vi "Toolbar Faacade.vi"(0 "Data In":T5, 2 "Display State In":T2={"Buttons Displayed"=0, "Button States"=[], "Button Size"=0, "Button Style"=enum."Classic", "Active Button"=0, "Force Regen?"=FALSE, "Tip String Ref"=refnum}, 3 "Container State":T4) -> (6 "Data Out":T5, 7 "Display State Out":T2={"Buttons Displayed"=0, "Button States"=[], "Button Size"=0, "Button Style"=enum."Classic", "Active Button"=0, "Force Regen?"=FALSE, "Tip String Ref"=refnum}, 8 "Action":T1)   [LabVIEW 2012, in "Toolbar.xctl"]
doc: "The business end of the XControl..."
uses:
  Toolbar.xctl
  Toolbar Data.ctl
  Button_Class/Type Defs/Button Events.ctl
  <vilib>/_xctls/Container State.ctl
  Toolbar State.ctl
  Button_Class/Button.lvclass
  Button_Class/Type Defs/Button Style.ctl
  <vilib>/_xctls/Action.ctl
  Button_Class/Type Defs/Button Status.ctl
  <vilib>/_xctls/XControlSupport.lvlib
panel:
  out "Display":picture[](array[picture])
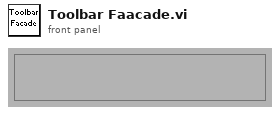
[diagram p1: front panel]
types:
  T1 = typedef "XControlSupport.lvlib/Action.ctl" = cluster{"Data Changed?":bool, "State Changed?":bool, "Action Name":string}
  T2 = typedef "Toolbar.xctl/Toolbar State.ctl" = cluster{"Buttons Displayed":i32, "Button States":refnum<class "Button.lvclass">[], "Button Size":i32, "Button Style":T3, "Active Button":i32, "Force Regen?":bool, "Tip String Ref":refnum<vi>}
  T3 = typedef "Button.lvclass/Button Style.ctl" = enum16{"System", "Modern", "Classic", "Rounded", "Silver", "Ni Theme", "Metallic"}
  T4 = typedef "XControlSupport.lvlib/Container State.ctl" = cluster{"Indicator?":bool, "Run Mode?":bool, " Refnum":refnum<vi>}
  T5 = typedef "Toolbar.xctl/Toolbar Data.ctl" = cluster{"Index":i32, "Type":T6}
  T6 = typedef "Button.lvclass/Button Events.ctl" = enum16{"Click", "Latch", "Unlatch"}
  T7 = typedef "Button.lvclass/Button Status.ctl" = enum16{"Off", "Hover", "On", "Disabled"}
  T8 = enum16{"NoButton", "Left Button", "Right Button", "Middle Button"}
  T9 = typedef "LVPoint32TypeDef.ctl" = cluster{"Horizontal":i32, "Vertical":i32}
  T10 = typedef "LVRectTypeDef.ctl" = cluster{"Left":i16, "Top":i16, "Right":i16, "Bottom":i16}
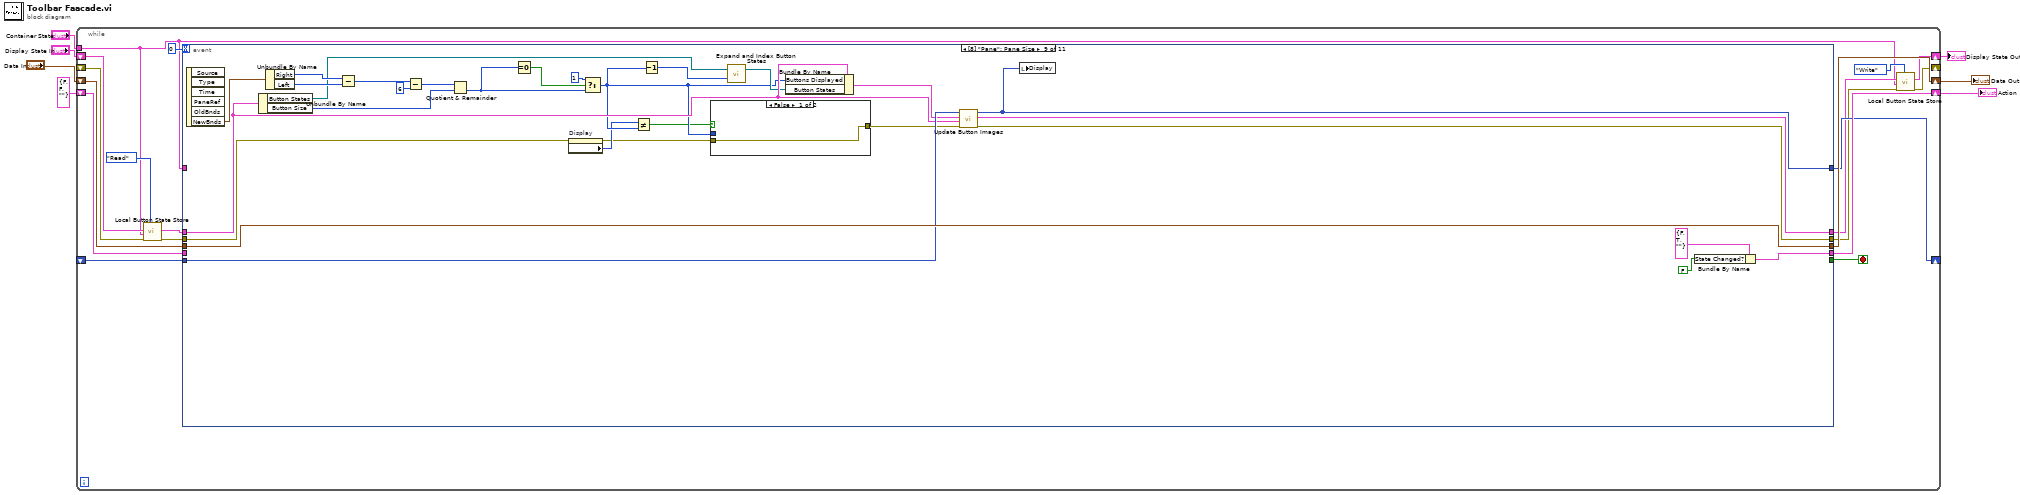
[diagram p0: block diagram]
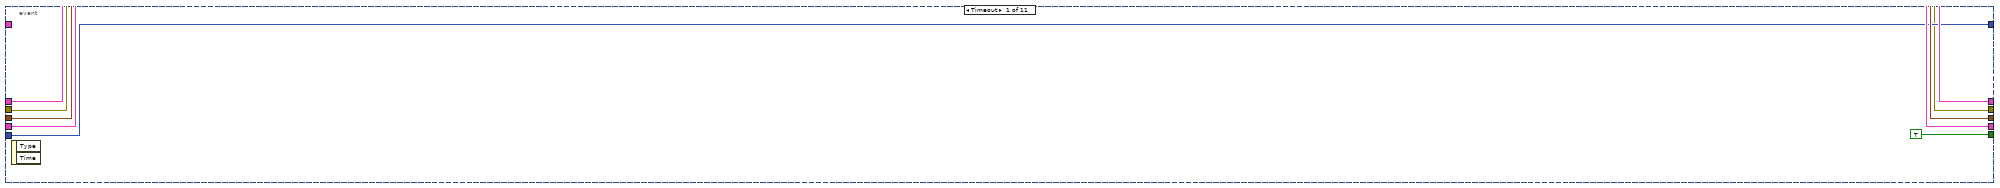
[diagram p2: hidden frame]
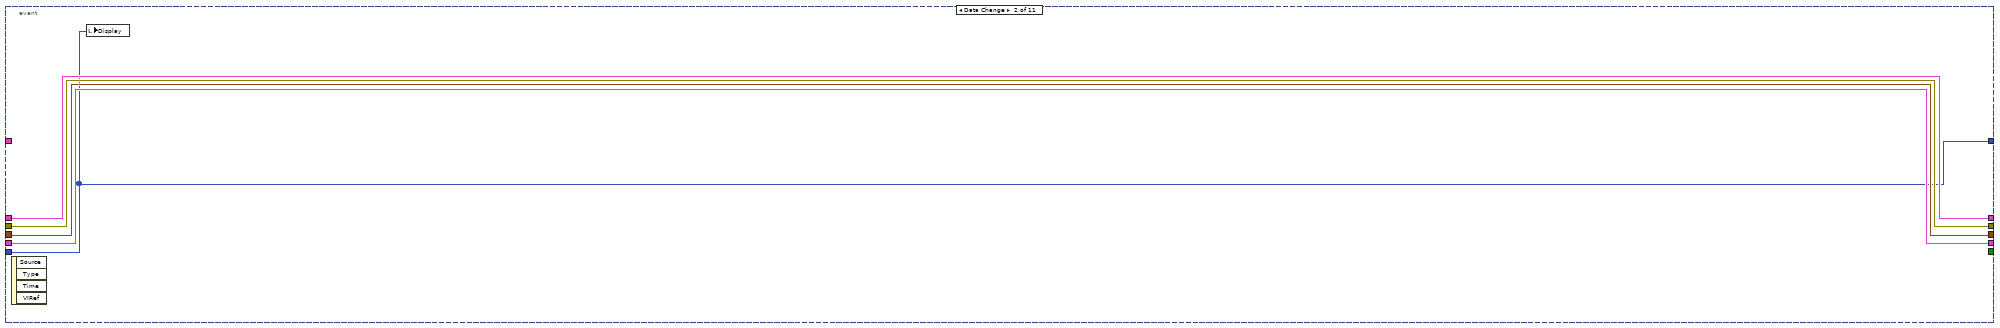
[diagram p3: hidden frame]
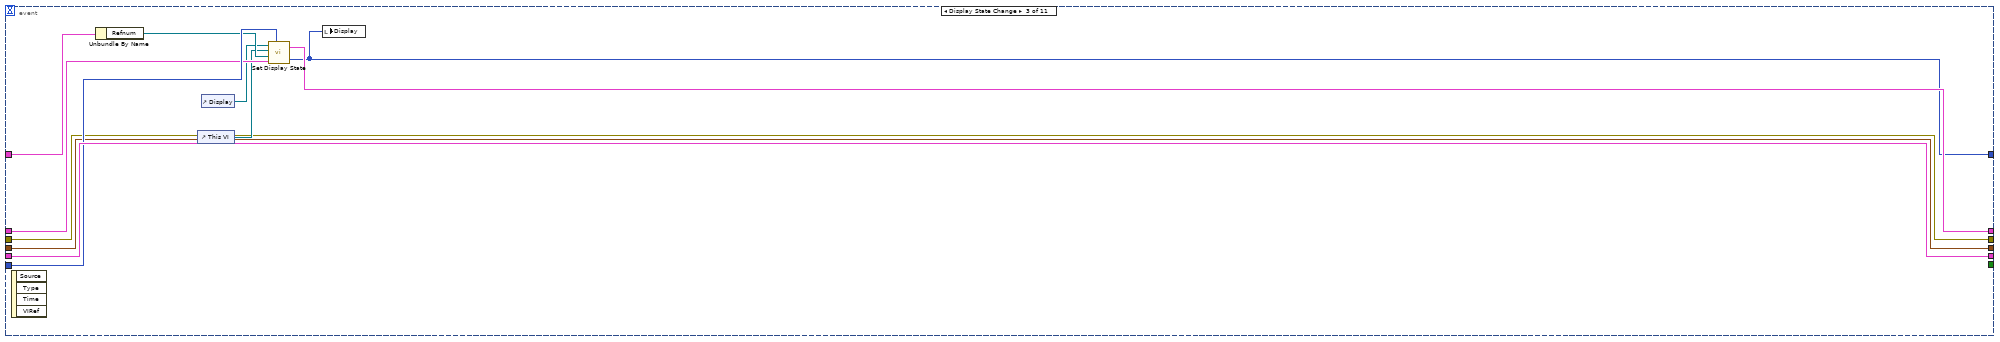
[diagram p4: hidden frame]
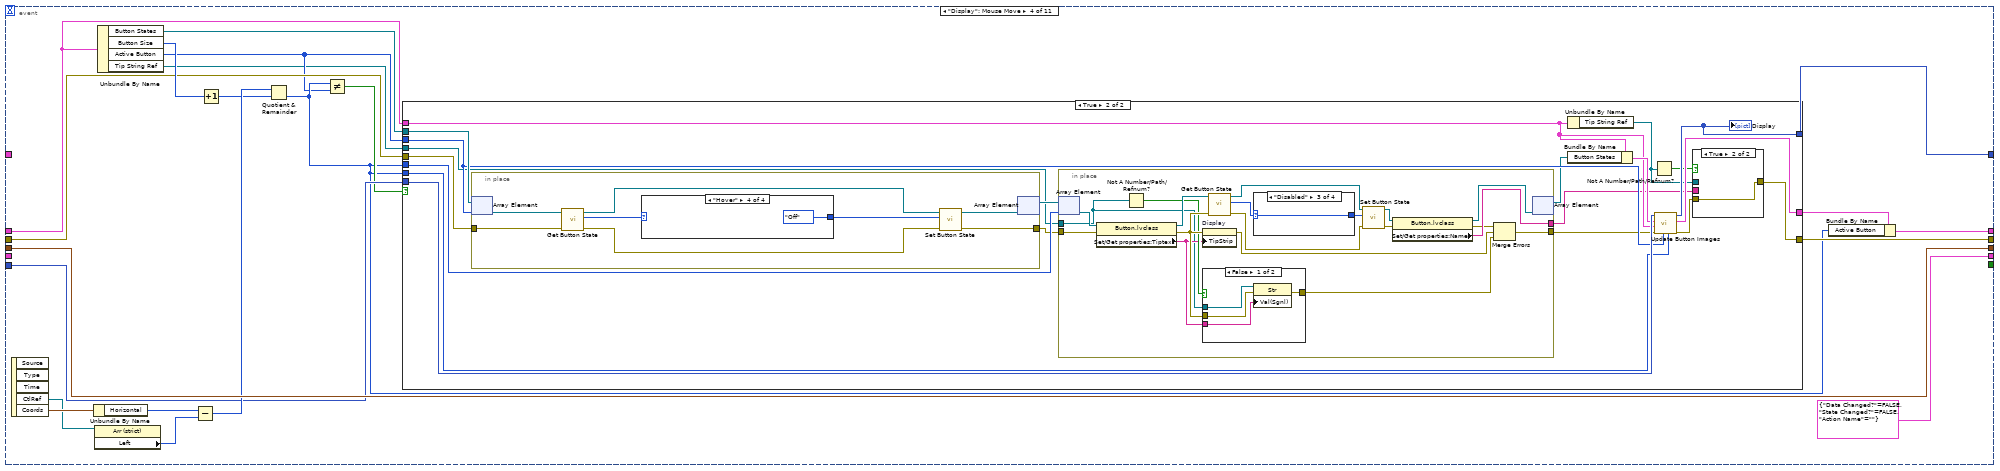
[diagram p5: hidden frame]
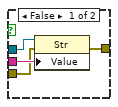
[diagram p7: hidden frame]
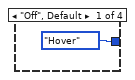
[diagram p9: hidden frame]
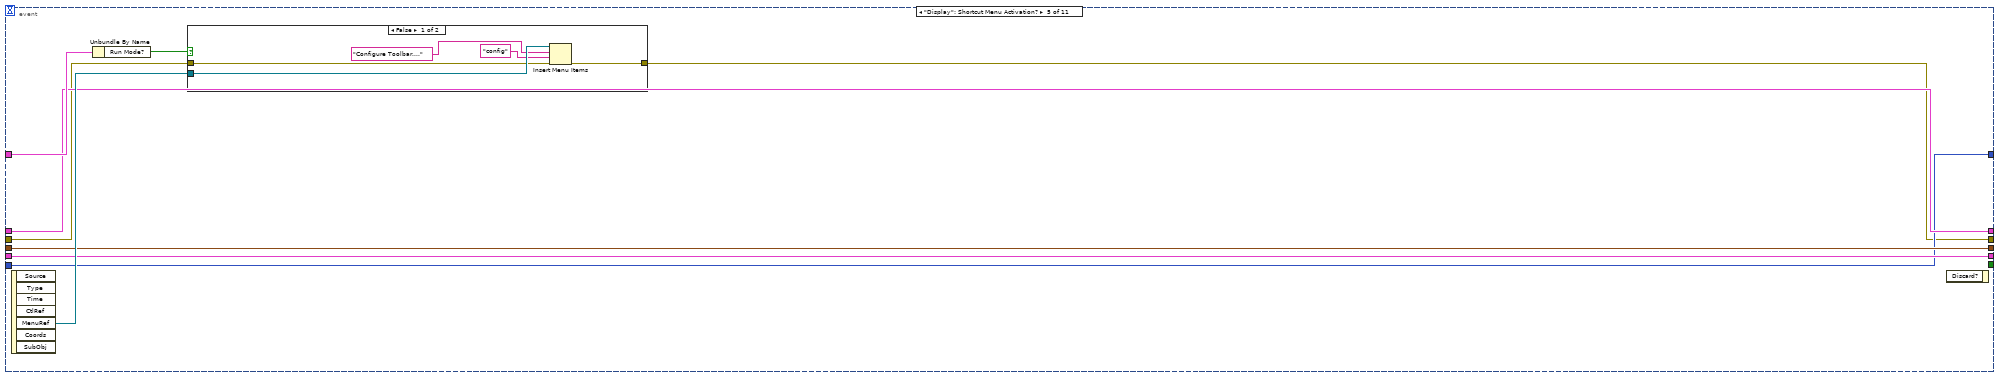
[diagram p15: hidden frame]
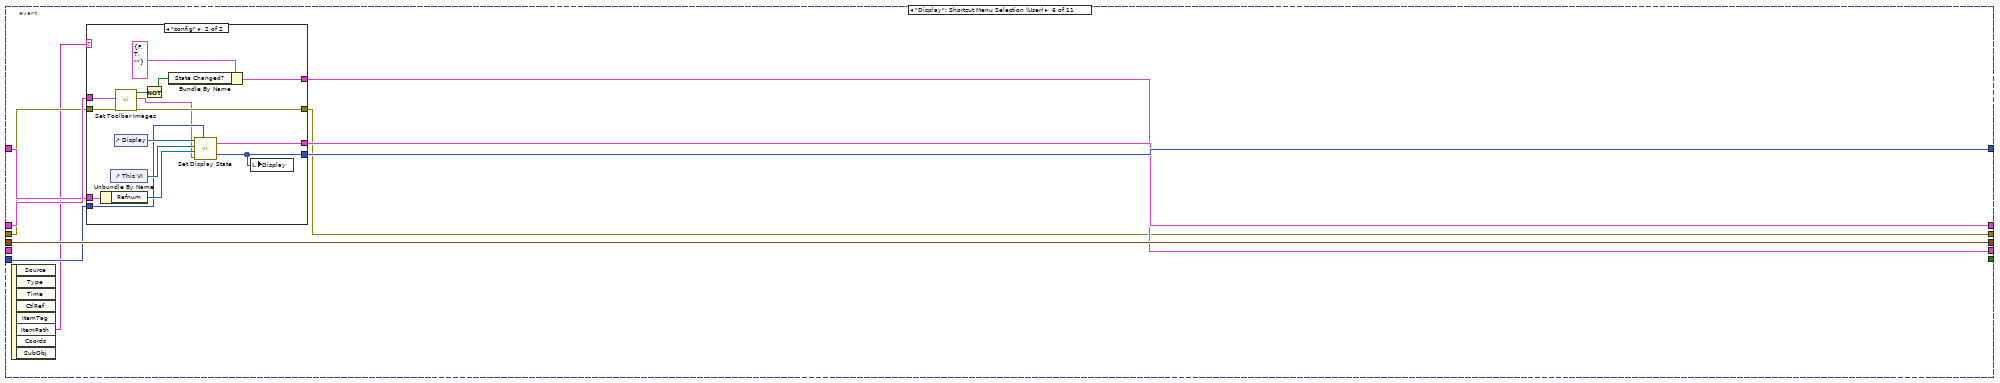
[diagram p17: hidden frame]
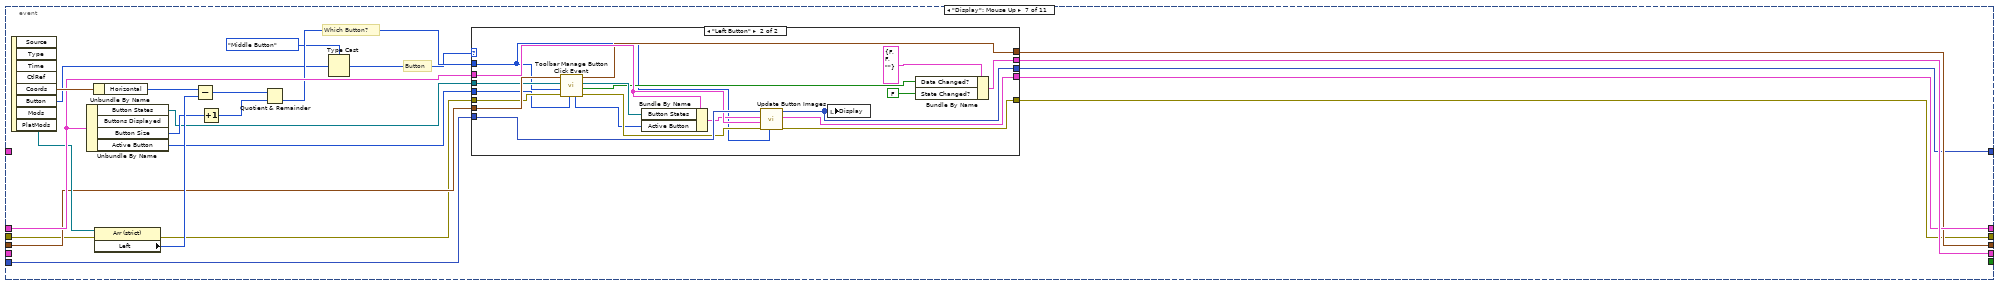
[diagram p19: hidden frame]
diagram:
  n1 = while {
    shift-right: [w8] -> w4
    shift-left: "Display State In" -> [w12]
    tunnel: "Container State" -> [w10]
    shift-right: [w23] -> w7
    shift-left: "Data In" -> [w24]
    shift-right: [w21] -> w2
    shift-left: T1 {"Data Changed?"=FALSE, "State Changed?"=FALSE, "Action Name"=""} ("Action") -> [w22]
    shift-right: [w20] -> _
    shift-left: _ -> [w19]
    shift-right: [w15] -> _
    shift-left: _ -> [w14]
    stop <- w26 stop-if-true
    n2 = call "Local Button State Store.vi"("Operation"=enum16{"Read", "Write"}."Read", "error in (no error)"=w14, "Container State"=w10, "Display State In"=w12) -> ("error out"=w13:errorcluster, "Display State Out"=w9:T2)  [unwired: 6 out]
    n3 = event shown="[8] \"Pane\": Pane Size" {
      selector: _ -> [_ _ _ _ _ _ _ _ _ _ _]
      dyn-events: _ -> [_ _ _ _ _ _ _ _ _ _ _]
      timeout: 0 -> [_ _ _ _ _ _ _ _ _ _ _]
      tunnel: w9 -> [w30 w36 w44 w53 w142 w161 w200 w230 w272 w295 w305]
      tunnel: [w30 w36 w41 w52 w142 w158 w195 w235 w270 w295 w304] -> w11
      tunnel: [TRUE _ _ _ _ _ _ _ _ _ _] -> w26
      tunnel: w10 -> [_ _ w46 _ w145 w157 _ _ _ w296 w311]
      tunnel: w24 -> [w29 w37 w39 w66 w143 w162 w193 w237 w278 w294 w310]
      tunnel: [w29 w37 w39 w66 w143 w162 w192 w237 w278 w294 w310] -> w23
      tunnel: [w31 w35 w48 T1 {"Data Changed?"=FALSE, "State Changed?"=FALSE, "Action Name"=""} ("Action") w141 w156 w203 T1 {"Data Changed?"=FALSE, "State Changed?"=FALSE, "Action Name"=""} ("Action") w263 w293 w309] -> w21
      tunnel: w22 -> [w31 w35 w48 _ w141 _ _ _ _ w293 w309]
      tunnel: [w28 w33 w38 w62 w140 w159 w191 w227 w256 w292 w307] -> w20
      tunnel: w19 -> [w28 w33 w47 w61 w140 w160 w190 w236 w276 w292 w308]
      tunnel: [w27 w34 w40 w57 w139 w154 w185 w232 w260 w288 w302] -> w16
      tunnel: w13 -> [w27 w34 w40 w56 w138 w155 w184 w234 w257 w289 w303]
      event Timeout {
        n4 = event-data() -> ()  [unwired: 3 out]
      }
      event Data Change {
        n5 = event-data() -> ()  [unwired: 5 out]
        n6 = local write "Display"(w33) -> ()
      }
      event Display State Change {
        n7 = event-data() -> ()  [unwired: 5 out]
        n8 = Unbundle By Name(w46) -> ("Refnum"=w45:refnum<vi>)
        n9 = control-ref of="This VI"() -> (w43:refnum<vi>)
        n10 = control-ref of="Display"() -> (w42:refnum<vi>)
        n11 = call "Set Display State.vi"("Picture Array Refnum"=w42, "Facade Vi Refnum"=w43, "Container Refnum"=w45, "Display State In"=w44, "Display"=w47) -> ("State Out"=w41:T2, "Images Out"=w38:picture[])
        n12 = local write "Display"(w38) -> ()
      }
      event "Display": Mouse Move {
        n13 = event-data() -> ("CtlRef"=w65:refnum<vi>, "Coords"=w68:T9)  [unwired: 4 out]
        n14 = Unbundle By Name(w68) -> ("Horizontal"=w67:i32)
        n15 = property class="Arr (strict)"(reference=w65) -> ("Left"=w63:i32)  [unwired: 1 in, 2 out]
        n16 = Unbundle By Name(w53) -> ("Button States"=w55:refnum<class "Button.lvclass">[], "Button Size"=w59:i32, "Active Button"=w50:i32, "Tip String Ref"=w49:refnum<vi>)
        n17 = Subtract(x=w67, y=w63) -> (x-y=w64:i32)
        n18 = Increment(x=w59) -> (x+1=w58:i32)
        n19 = Quotient & Remainder(x=w64, y=w58) -> (floor(x/y)=w51:i32)  [unwired: 1 out]
        n20 = Not Equal?(x=w51, y=w50) -> (x != y?=w54:bool)
        n21 = case shown="True" w54 {
          tunnel: [w72 w80] -> w62
          tunnel: w61 -> [w72 w92]
          tunnel: w53 -> [w71 w79]
          tunnel: [w71 w90] -> w60
          tunnel: [w70 w74] -> w57
          tunnel: w56 -> [w70 w86]
          tunnel: w55 -> [_ w88]
          tunnel: w51 -> [_ w84]
          tunnel: w50 -> [_ w87]
          tunnel: w51 -> [_ w89]
          tunnel: w49 -> [_ w73]
          frame False {
          }
          frame True {
            n22 = in-place {
              in-place-border: w86 -> [w129]
              in-place-border: [w126] -> w83
              n23 = in-place-array #1(w88, w87) -> (w133:refnum<class "Button.lvclass">)
              n24 = call-dynamic "Get Button State.vi"("error in (no error)"=w129, "Button in"=w133) -> ("error out"=w128:errorcluster, "State"=w131:T7, "Button out"=w132:refnum<class "Button.lvclass">)  [unwired: 1 in, 6 out]
              n25 = case shown="\"Hover\"" w131 {
                selector: w131 -> [w134 w135 w136 _]
                tunnel: [w134 w135 w136 Button_Status."Off" ("State")] -> w130
                frame "Off", Default {
                }
                frame "On" {
                }
                frame "Disabled" {
                }
                frame "Hover" {
                }
              }
              n26 = call-dynamic "Set Button State.vi"("error in (no error)"=w128, "State"=w130, "Button in"=w132) -> ("error out"=w126:errorcluster, "Button out"=w127:refnum<class "Button.lvclass">)  [unwired: 7 out]
              n27 = in-place-array #1(w127) -> (w85:refnum<class "Button.lvclass">[])  [unwired: 1 out]
            }
            n28 = in-place {
              in-place-border: w83 -> [w107]
              in-place-border: [w99] -> w81
              in-place-border: [w109] -> w76
              in-place-border: w73 -> [w98]
              n29 = in-place-array #2(w85, w84) -> (w116:refnum<class "Button.lvclass">)
              n30 = property class="Button.lvclass"(reference=w116, error in=w107) -> (reference out=w108:refnum<class "Button.lvclass">, error out=w106:errorcluster, "Set/Get properties:Tiptext"=w104:string)
              n31 = Not A Number/Path/Refnum?(number/path/refnum=w98) -> (NaN/Path/Refnum?=w105:bool)
              n32 = property on="Display" class="Arr (strict)"(error in=w106, "TipStrip"=w104) -> (error out=w101:errorcluster)  [unwired: 1 in, 1 out]
              n33 = case shown="False" w105 {
                tunnel: w106 -> [w120 w121]
                tunnel: w104 -> [w119 _]
                tunnel: [w118 w121] -> w100
                tunnel: w98 -> [w117 _]
                frame False {
                  n34 = property class="Str"(reference=w117, error in=w120, "Val(Sgnl)"=w119) -> (error out=w118:errorcluster)  [unwired: 1 out]
                }
                frame True {
                }
              }
              n35 = call-dynamic "Get Button State.vi"("error in (no error)"=w106, "Button in"=w108) -> ("error out"=w112:errorcluster, "State"=w114:T7, "Button out"=w115:refnum<class "Button.lvclass">)  [unwired: 1 in, 6 out]
              n36 = case shown="\"Disabled\"" w114 {
                selector: w114 -> [_ w123 w124 w125]
                tunnel: [Button_Status."Hover" ("State") w123 w124 w125] -> w113
                frame "Off", Default {
                }
                frame "On" {
                }
                frame "Disabled" {
                }
                frame "Hover" {
                }
              }
              n37 = call-dynamic "Set Button State.vi"("error in (no error)"=w112, "State"=w113, "Button in"=w115) -> ("error out"=w103:errorcluster, "Button out"=w111:refnum<class "Button.lvclass">)  [unwired: 7 out]
              n38 = property class="Button.lvclass"(reference=w111, error in=w103) -> (reference out=w110:refnum<class "Button.lvclass">, error out=w102:errorcluster, "Set/Get properties:Name"=w109:string)
              n39 = Merge Errors(w102, w101, w100) -> (w99:errorcluster)
              n40 = in-place-array #2(w110) -> (w82:refnum<class "Button.lvclass">[])  [unwired: 1 out]
            }
            n41 = Unbundle By Name(w79) -> ("Tip String Ref"=w77:refnum<vi>)
            n42 = Bundle By Name(cluster=w79, "Button States"=w82) -> (w91:T2)
            n43 = Not A Number/Path/Refnum?(number/path/refnum=w77) -> (NaN/Path/Refnum?=w78:bool)
            n44 = call "Update Button Images.vi"("New Index"=w89, "Old Index"=w87, "error in (no error)"=w81, "Old State"=w79, "New State"=w91, "Images In"=w92) -> ("error out"=w75:errorcluster, "State Out"=w90:T2, "Images Out"=w80:picture[])  [unwired: 1 in, 2 out]
            "Display" <- w80
            n45 = case shown="True" w78 {
              tunnel: w77 -> [w96 _]
              tunnel: w76 -> [w95 _]
              tunnel: w75 -> [w94 w97]
              tunnel: [w93 w97] -> w74
              frame False {
                n46 = property class="Str"(reference=w96, error in=w94, "Value"=w95) -> (error out=w93:errorcluster)  [unwired: 1 out]
              }
              frame True {
              }
            }
          }
        }
        n47 = Bundle By Name(cluster=w60, "Active Button"=w51) -> (w52:T2)
      }
      event "Display": Shortcut Menu Activation? {
        n48 = event-data() -> ("MenuRef"=w146:refnum<k9>)  [unwired: 7 out]
        n49 = Unbundle By Name(w145) -> ("Run Mode?"=w144:bool)
        n50 = case shown="False" w144 {
          tunnel: w146 -> [w151 _]
          tunnel: [w148 w152] -> w139
          tunnel: w138 -> [w147 w152]
          frame False {
            n51 = Insert Menu Items(6:w147, 7:"config" ("item tags"), 8:"Configure Toolbar....", 9:w151) -> (0:w148:errorcluster)  [unwired: 4 out]
          }
          frame True {
          }
        }
        n52 = event-data() -> ()  [unwired: 1 in, 2 out]
      }
      event "Display": Shortcut Menu Selection (User) {
        n53 = event-data() -> ("ItemPath"=w153:string)  [unwired: 8 out]
        n54 = case shown="\"config\"" w153 {
          tunnel: w161 -> [w165 w179]
          tunnel: w160 -> [w163 w171]
          tunnel: [w163 w172] -> w159
          tunnel: [w165 w176] -> w158
          tunnel: w157 -> [_ w175]
          tunnel: [_ w173] -> w156
          tunnel: w155 -> [w164 w170]
          tunnel: [w164 w169] -> w154
          frame "False", Default {
          }
          frame "config" {
            n55 = Unbundle By Name(w175) -> ("Refnum"=w174:refnum<vi>)
            n56 = control-ref of="This VI"() -> (w178:refnum<vi>)
            n57 = control-ref of="Display"() -> (w177:refnum<vi>)
            n58 = call "Set Toolbar Images.vi"("error in (no error)"=w170, "State"=w179) -> ("error out"=w169:errorcluster, "State Out"=w166:T2, "Cancelled?"=w168:bool)  [unwired: 7 out]
            n59 = Not(x=w168) -> (.not. x?=w167:bool)
            n60 = Bundle By Name(cluster=T1 {"Data Changed?"=FALSE, "State Changed?"=TRUE, "Action Name"=""} ("Action"), "State Changed?"=w167) -> (w173:T1)
            n61 = call "Set Display State.vi"("Picture Array Refnum"=w177, "Facade Vi Refnum"=w178, "Container Refnum"=w174, "Display State In"=w166, "Display"=w171) -> ("State Out"=w176:T2, "Images Out"=w172:picture[])
            n62 = local write "Display"(w172) -> ()
          }
        }
      }
      event "Display": Mouse Up {
        # "Which Button?"
        # "Button"
        n63 = event-data() -> ("CtlRef"=w198:refnum<vi>, "Coords"=w202:T9, "Button"=w194:u16)  [unwired: 6 out]
        n64 = Unbundle By Name(w200) -> ("Button States"=w181:refnum<class "Button.lvclass">[], "Button Size"=w189:i32, "Active Button"=w182:i32)  [unwired: 1 out]
        n65 = Unbundle By Name(w202) -> ("Horizontal"=w201:i32)
        n66 = property class="Arr (strict)"(reference=w198, error in=w184) -> (error out=w183:errorcluster, "Left"=w196:i32)  [unwired: 1 out]
        n67 = Subtract(x=w201, y=w196) -> (x-y=w197:i32)
        n68 = Increment(x=w189) -> (x+1=w188:i32)
        n69 = Quotient & Remainder(x=w197, y=w188) -> (floor(x/y)=w199:i32)  [unwired: 1 out]
        n70 = Type Cast(type=T8."Middle Button", x=w194) -> (*(type *) &x=w187:T8)
        n71 = case shown="\"Left Button\"" w187 {
          tunnel: [_ w224] -> w203
          tunnel: w181 -> [_ w214]
          tunnel: w200 -> [w207 w221]
          tunnel: w199 -> [_ w211]
          tunnel: [w207 w219] -> w195
          tunnel: w193 -> [w206 w226]
          tunnel: [w206 w215] -> w192
          tunnel: [w205 w208] -> w191
          tunnel: w190 -> [w205 w222]
          tunnel: [w204 w217] -> w185
          tunnel: w183 -> [w204 w216]
          tunnel: w182 -> [_ w210]
          frame "NoButton", Default {
          }
          frame "Left Button" {
            n72 = call "Toolbar Manage Button Click Event.vi"("Index In"=w210, "error in (no Error)"=w216, "Button Index"=w211, "Button States In"=w214, "Data In"=w226) -> ("error out"=w218:errorcluster, "Data Changed ?"=w212:bool, "Button States Out"=w213:refnum<class "Button.lvclass">[], "Data Out"=w215:T5, "Index Out"=w209:i32)  [unwired: 2 out]
            n73 = Bundle By Name(cluster=w221, "Button States"=w213, "Active Button"=w209) -> (w220:T2)
            n74 = call "Update Button Images.vi"("Old Index"=w211, "error in (no error)"=w218, "Old State"=w221, "New State"=w220, "Images In"=w222) -> ("error out"=w217:errorcluster, "State Out"=w219:T2, "Images Out"=w208:picture[])  [unwired: 2 in, 2 out]
            n75 = local write "Display"(w208) -> ()
            n76 = Bundle By Name(cluster=T1 {"Data Changed?"=FALSE, "State Changed?"=FALSE, "Action Name"=""} ("Action"), "Data Changed?"=w212, "State Changed?"=FALSE) -> (w224:T1)
          }
        }
      }
      event "Display": Mouse Leave {
        n77 = event-data() -> ()  [unwired: 5 out]
        n78 = in-place {
          in-place-border: w230 -> [_]
          in-place-border: w234 -> [w244]
          in-place-border: [w243] -> w233
          in-place-border: [w239] -> w231
          w239 = -1
          n79 = in-place-cluster #3(w230) -> ("Button States"=w242:refnum<class "Button.lvclass">[], "Active Button"=w241:i32)
          n80 = in-place {
            in-place-border: w244 -> [w252]
            in-place-border: [w251] -> w243
            n81 = in-place-array #4(w242, w241) -> (w246:refnum<class "Button.lvclass">)
            n82 = call-dynamic "Get Button State.vi"("error in (no error)"=w252, "Button in"=w246) -> ("error out"=w247:errorcluster, "State"=w248:T7, "Button out"=w249:refnum<class "Button.lvclass">)  [unwired: 7 out]
            n83 = case shown="\"Hover\"" w248 {
              selector: w248 -> [w253 _]
              tunnel: [w253 Button_Status."Off" ("State")] -> w250
              frame "Off", Default {
              }
              frame "Hover" {
              }
            }
            n84 = call-dynamic "Set Button State.vi"("error in (no error)"=w247, "State"=w250, "Button in"=w249) -> ("error out"=w251:errorcluster, "Button out"=w245:refnum<class "Button.lvclass">)  [unwired: 7 out]
            n85 = in-place-array #4(w245) -> (w240:refnum<class "Button.lvclass">[])  [unwired: 1 out]
          }
          n86 = in-place-cluster #3("Button States"=w240, "Active Button"=w239) -> (w229:T2)
        }
        n87 = call "Update Button Images.vi"("New Index"=w231, "Force Regen"=FALSE, "error in (no error)"=w233, "Old State"=w230, "New State"=w229, "Images In"=w236) -> ("error out"=w232:errorcluster, "State Out"=w235:T2, "Images Out"=w227:picture[])  [unwired: 1 in, 2 out]
        n88 = local write "Display"(w227) -> ()
      }
      event Pane Size {
        n89 = event-data() -> ("NewBnds"=w264:T10)  [unwired: 6 out]
        n90 = Unbundle By Name(w272) -> ("Button States"=w255:refnum<class "Button.lvclass">[], "Button Size"=w269:i32)
        n91 = Unbundle By Name(w264) -> ("Right"=w283:i16, "Left"=w282:i16)
        n92 = Subtract(x=w283, y=w282) -> (x-y=w274:i16)
        n93 = Subtract(x=w274, y=i16 6) -> (x-y=w275:i16)
        n94 = Quotient & Remainder(x=w275, y=w269) -> (floor(x/y)=w281:i32)  [unwired: 1 out]
        n95 = Equal To 0?(x=w281) -> (x = 0?=w277:bool)
        n96 = property on="Display" class="Arr (strict)"(error in=w257) -> (error out=w258:errorcluster, "Number of Columns"=w265:u32)  [unwired: 1 in, 1 out]
        n97 = Select(t=i16 1, s=w277, f=w281) -> (s? t:f=w266:i32)
        n98 = Not Equal?(x=w265, y=w266) -> (x != y?=w262:bool)
        n99 = Decrement(x=w266) -> (x-1=w267:i32)
        n100 = case shown="False" w262 {
          tunnel: w266 -> [_ w287]
          tunnel: [w284 w286] -> w259
          tunnel: w258 -> [w284 w285]
          frame False {
          }
          frame True {
            n101 = property on="Display" class="Arr (strict)"(error in=w285, "Number of Columns"=w287) -> (error out=w286:errorcluster)  [unwired: 1 in, 1 out]
          }
        }
        n102 = call "Expand and Index Button States.vi"("Button Index"=w267, "Button States"=w255) -> ("Button States Out"=w268:refnum<class "Button.lvclass">[])  [unwired: 1 out]
        n103 = Bundle By Name(cluster=w272, "Buttons Displayed"=w266, "Button States"=w268) -> (w271:T2)
        n104 = call "Update Button Images.vi"("error in (no error)"=w259, "Old State"=w272, "New State"=w271, "Images In"=w276) -> ("error out"=w260:errorcluster, "State Out"=w270:T2, "Images Out"=w256:picture[])  [unwired: 3 in, 2 out]
        n105 = local write "Display"(w256) -> ()
        n106 = Bundle By Name(cluster=T1 {"Data Changed?"=FALSE, "State Changed?"=TRUE, "Action Name"=""} ("Action"), "State Changed?"=FALSE) -> (w263:T1)
      }
      event Direction Change {
        n107 = event-data() -> ()  [unwired: 5 out]
        n108 = Unbundle By Name(w296) -> ("Indicator?"=w290:bool, "Refnum"=w291:refnum<vi>)
        n109 = case shown="True" w290 {
          tunnel: w291 -> [_ w301]
          tunnel: w289 -> [w297 w299]
          tunnel: [w297 w298] -> w288
          frame False {
          }
          frame True {
            # "The direction of the XControl changed from a control to an indicator or vice versa. Update the appearance accordingly."
            n110 = property class="Ctl"(reference=w301, error in=w299, "Indicator"=FALSE) -> (error out=w298:errorcluster)  [unwired: 1 out]
          }
        }
      }
      event Exec State Change {
        n111 = event-data() -> ()  [unwired: 5 out]
        n112 = Unbundle By Name(w311) -> ("Run Mode?"=w306:bool)
        n113 = call "Update Button Images.vi"("Force Regen"=w306, "error in (no error)"=w303, "Old State"=w305, "New State"=w305, "Images In"=w308) -> ("error out"=w302:errorcluster, "State Out"=w304:T2, "Images Out"=w307:picture[])  [unwired: 2 in, 2 out]
        n114 = local write "Display"(w307) -> ()
      }
    }
    n115 = call "Local Button State Store.vi"("Operation"=enum16{"Read", "Write"}."Write", "error in (no error)"=w16, "Container State"=w10, "Display State In"=w11) -> ("error out"=w15:errorcluster, "Display State Out"=w8:T2)  [unwired: 1 in, 5 out]
  }
  "Display State Out" <- w4
  "Data Out" <- w7
  "Action" <- w2
